vi "LOAD CELL READ.vi"(8 "error in (no error)":errorcluster, 11 "main ref":T1) -> (0 "error out":errorcluster)   [LabVIEW 2025]
uses:
  controls/LAB-IQ UI Data.ctl
  <vilib>/Analysis/baseanly.llb/Mean (DBL).vi
  <vilib>/Analysis/5stat.llb/RMS (DBL).vi
  <vilib>/Analysis/NI_AALBase.lvlib
  <vilib>/ptbypt/NI_PtbyPt.lvlib
  <vilib>/Analysis/NI_AALPro.lvlib
panel:
  out "Fload 3":dbl
  out "Fload 2":dbl
  out "Fload":dbl
  out "Friction":dbl
  out "Load Temp":dbl
  out "Zload":dbl
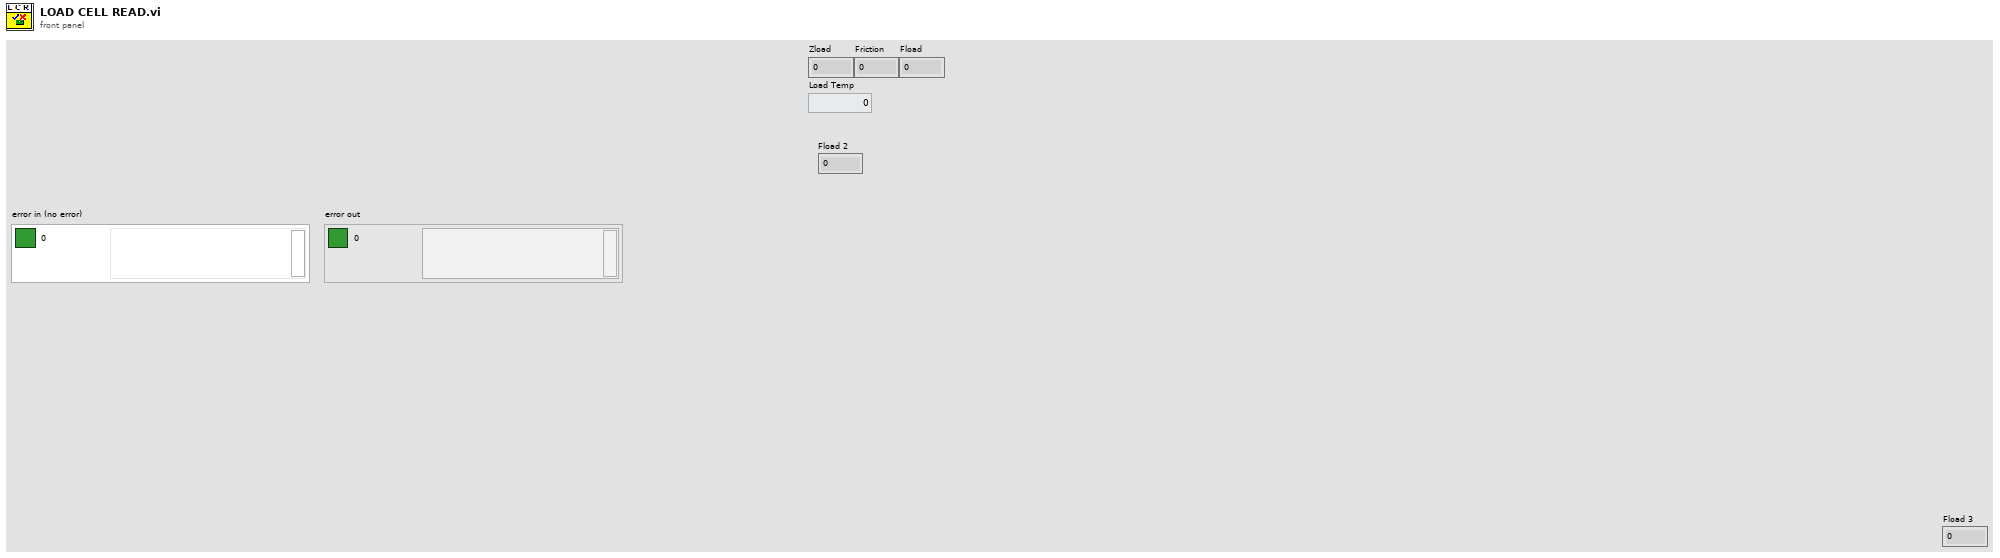
[diagram p1: front panel]
types:
  T1 = typedef "LAB-IQ UI Data.ctl" = cluster{"Main Home Screen":cluster{"GUI":refnum<vi>, "Platform Settings":refnum<vi>, "Configure":refnum<vi>, "Home":refnum<vi>, "EXIT":refnum<vi>, "service 2":refnum<vi>, "MainPage":refnum<vi>, "Analysis":refnum<vi>}, "Platform Settings":cluster{"mm/s  Surge":refnum<vi>, "Update Surge Speed":refnum<vi>, "Drive Error":refnum<vi>, "Disable Axis Jog Soft Limits":refnum<vi>, "mm/s  Sway":refnum<vi>, "Sway and Surge COM Status":refnum<vi>, "Heave COM Status":refnum<vi>, "Enable Platform":refnum<vi>, "Surge Forward Main":refnum<vi>, "Sway Right Main":refnum<vi>, "Sway Left Main":refnum<vi>, "Heave Down Main":refnum<vi>, "Heave Up main":refnum<vi>, "Update Sway Speed":refnum<vi>, "Update Heave Speed":refnum<vi>, "mm/s Heave":refnum<vi>, "mm/sec":refnum<vi>, "mm":refnum<vi>, "Surge Backward Main":refnum<vi>}, "Analysis Screen":cluster{"Analysis Home":refnum<vi>, "Surface Analysis":refnum<vi>, "Imaging":refnum<vi>, "Image Analysis":refnum<vi>, "Post Analysis":refnum<vi>}, "Config Screen":cluster{"Select Load Head":refnum<vi>, "Notes :":refnum<vi>, "FILE":refnum<vi>, "Sample ID :":refnum<vi>, "Operator ID :":refnum<vi>, "Operator Name :":refnum<vi>, "Auto":refnum<vi>}, "Motion Module":cluster{"zNL":refnum<vi>, "NL disp":refnum<vi>, "Rotary Tab":refnum<vi>, "Motion Direction:  3":refnum<vi>, "E.Velocity 2":refnum<vi>, "e.v/ssr 2":refnum<vi>, "Enter Fixed E.Velocity 2":refnum<vi>, "Enter Final SRR 2":refnum<vi>, "Enter initial SRR 2":refnum<vi>, "Enter Fixed SRR 2":refnum<vi>, "Enter the Final E.Velocity (m/s) 2":refnum<vi>, "Enter initial E.Velocity (m/s) 2":refnum<vi>, "Final Speed (RPM) 3":refnum<vi>, "Initial Speed (RPM) 2":refnum<vi>, "Enter the Final Velocity (m/s) 3":refnum<vi>, "Enter initial Velocity (m/s)  3":refnum<vi>, "Ramp Up 2":refnum<vi>, "TEST SELECTION":refnum<vi>, "SPEED SELECTION : ":refnum<vi>, "Angular Oscillation Set":refnum<vi>, "Traction":refnum<vi>, "Step Speed":refnum<vi>, "StepTable For Load-Speed":refnum<vi>, "StepTable For Speed":refnum<vi>, "Surge Forward MM":refnum<vi>, "Surge Backward MM":refnum<vi>, "M3 Image":refnum<vi>, "String 39":refnum<vi>, "Sway Left MM":refnum<vi>, "Sway Right MM":refnum<vi>, "Disable Axis Jog Soft Limits":refnum<vi>, "mm":refnum<vi>, "Heave Down MM":refnum<vi>, "Heave Up MM":refnum<vi>, "Wear Track Diameter (mm)":refnum<vi>, "Set WTD":refnum<vi>, "HomeScratch":refnum<vi>, "HomeRot":refnum<vi>, "PlaceModule":refnum<vi>, "Enter the Angle (Deg)":refnum<vi>, "Enter the Frequency (Hz)":refnum<vi>, "Motion Mode:":refnum<vi>, "LR Sway":refnum<vi>, "Rot Hor":refnum<vi>, "Scratch":refnum<vi>, "LR Cam":refnum<vi>, "MMBack":refnum<vi>, "MMNext":refnum<vi>, "Rot Ver":refnum<vi>, "Rotary Module Selection":refnum<vi>, "calculate rotary":refnum<vi>, "SPEED SELECTION : rotary":refnum<vi>, "Import 2":refnum<vi>, "Save 2":refnum<vi>, "File Path :  2":refnum<vi>, "String 45":refnum<vi>, "StepTable For Speed 3":refnum<vi>, "Enter the Speed(mm/sec)":refnum<vi>, "Enter the Speed(RPM)":refnum<vi>, "Enter Scratch Speed (mm/s):":refnum<vi>, "SwaySpeed Set":refnum<vi>, "Scartch Offset":refnum<vi>, "Motion type:":refnum<vi>, "HomeScratch 2":refnum<vi>, "Enter Scratch length (mm):":refnum<vi>, "Wear Track Diameter":refnum<vi>, "Rotary Speed Exced":refnum<vi>, "Scratch Mode":refnum<vi>, "No of Scratch":refnum<vi>}, "Environmental control":cluster{"Humidity  Status  3":refnum<vi>, "Low Temp  Status  2":refnum<vi>, "TK4 status 2":refnum<vi>, "Stage Temperature":refnum<vi>, "Sample Temperature":refnum<vi>, "Humidity (Amb)":refnum<vi>, "Clear List":refnum<vi>, "Add to list":refnum<vi>, "Wear":refnum<vi>, "Vibration":refnum<vi>, "Humidity (Chamber)":refnum<vi>, "Temperature (Chamber)":refnum<vi>, "ECR ":refnum<vi>, "Temperature (Amb)":refnum<vi>, "Microphone":refnum<vi>, "Acoustic Emission 3":refnum<vi>, "SNext":refnum<vi>, "APBack":refnum<vi>, "Enter the Temperature (°C):":refnum<vi>, "Enter the Stage \nTemperature (°C):":refnum<vi>, "Enter the Humidity (%Rh):":refnum<vi>, "Low Temp":refnum<vi>, "High Temp":refnum<vi>, "Humidity":refnum<vi>, "Sensors Picked":refnum<vi>}, "About Screen":cluster{"Password":refnum<vi>, "Home Service":refnum<vi>, "Advanced Setting":refnum<vi>, "About Tab":refnum<vi>, "ECR Port:":refnum<vi>, "Ramp Port:":refnum<vi>, "Installation/Replacement completed":refnum<vi>, "Loahead":refnum<vi>, "Heave and Surge COM Port:":refnum<vi>, "Sway COM Port:":refnum<vi>, "Temp Modbus:":refnum<vi>, "Humidity Port:":refnum<vi>, "Edit Gain Constants":refnum<vi>, "Save Gain Constants":refnum<vi>}, "Main Screen":cluster{"Main Screen Tab":refnum<vi>, "Angle and Frequency":refnum<vi>, "Stroke (mm)":refnum<vi>, "Angle (Deg)":refnum<vi>, "Main Speed Tab":refnum<vi>, "MTM MOTOR DISPLAY":refnum<vi>, "Disc Speed (m/sec)":refnum<vi>, "Ball Speed (m/sec)":refnum<vi>, "Disc Speed (RPM)":refnum<vi>, "Ball Speed (RPM)":refnum<vi>, "SPEED TAB":refnum<vi>, "Speed (m/sec)":refnum<vi>, "Set Speed (m/sec)":refnum<vi>, "Speed (RPM)":refnum<vi>, "Set Speed":refnum<vi>, "Time Tab":refnum<vi>, "Time ( HH:MM:SS ) 2":refnum<vi>, "Test Duration":refnum<vi>, "Test Duration 4":refnum<vi>, "TEST CYCLE":refnum<vi>, "TOTAL CYCLES":refnum<vi>, "Set Load (N)":refnum<vi>, "Temp Tabs":refnum<vi>, "Heater":refnum<vi>, "TK4 status":refnum<vi>, "ChamberTemp":refnum<vi>, "SetTmp":refnum<vi>, "Controller  Status":refnum<vi>, "ChamberTemp 2":refnum<vi>, "SetTmp 2":refnum<vi>, "Controller  Status 2":refnum<vi>, "ChamberTemp 3":refnum<vi>, "SetTmp 3":refnum<vi>, "Cooling":refnum<vi>, "Load Communication":refnum<vi>, "Ambient \nTemperature":refnum<vi>, "HumCOMStatus":refnum<vi>, "Ambient\n Humidity":refnum<vi>, "Freq (Hz)":refnum<vi>, "Load En":refnum<vi>, "NLt":refnum<vi>, "zNL 2":refnum<vi>, "Humidity On":refnum<vi>, "humidity disp":refnum<vi>, "Set Humidity":refnum<vi>, "NL disp 2":refnum<vi>, "Humidity On 2":refnum<vi>, "humidity disp 2":refnum<vi>, "Set Humidity 2":refnum<vi>, "NL disp 3":refnum<vi>, "AppLoadSeq scratch":refnum<vi>, "Stop Scratch":refnum<vi>, "ClrLog":refnum<vi>, "Trip Log":refnum<vi>, "STOP":refnum<vi>, "Start Test":refnum<vi>, "Test status":refnum<vi>, "AR Led":refnum<vi>, "Data":refnum<vi>, "Health":refnum<vi>, "Sway COM Status":refnum<vi>, "Heave COM Status":refnum<vi>, "Grp Tab":refnum<vi>, "Sub Graph":refnum<vi>, "SD (mm)":refnum<vi>, "Siliding distance Reset Graph":refnum<vi>, "SDGp":refnum<vi>, "Humidity Reset Graph":refnum<vi>, "HumrGp":refnum<vi>, "Acoustic Emission (mV)":refnum<vi>, "Aqucostic Reset Graph":refnum<vi>, "gACQUOS":refnum<vi>, "ECR RESET":refnum<vi>, "ECR":refnum<vi>, "Temperature Reset":refnum<vi>, "Acoustic Emission (mV) 2":refnum<vi>, "Aqucostic Reset Graph 2":refnum<vi>, "gACQUOS 2":refnum<vi>, "ECR RESET 2":refnum<vi>, "ECR 2":refnum<vi>, "Temperature Reset 2":refnum<vi>, "Temperature (deg c)":refnum<vi>, "Speed Reset Graph":refnum<vi>, "Speed Tab":refnum<vi>, "MTM DISC  SPEED":refnum<vi>, "MTM BALL SPEED":refnum<vi>, "speed mm/sec":refnum<vi>, "Hymidity":refnum<vi>, "Humidity Disable trip":refnum<vi>, "CoF Trip  2":refnum<vi>, "Depth Trip":refnum<vi>, "Weart Deapth":refnum<vi>, "Depth Reset Graph":refnum<vi>, "Weart":refnum<vi>, "Depthz":refnum<vi>, "Depth (µm)":refnum<vi>, "WearGp":refnum<vi>, "NL Trip 2":refnum<vi>, "Load pid":refnum<vi>, "Load Disable Trip":refnum<vi>, "Load Reset Graph":refnum<vi>, "NL Display 4":refnum<vi>, "Main Chart 3":refnum<vi>, "BACK":refnum<vi>, "Depth Trip 2":refnum<vi>, "COF TRIP ":refnum<vi>, "Friction Force (N)":refnum<vi>, "FF Reset Graph":refnum<vi>, "FF Disable Trip":refnum<vi>, "FF TRIP":refnum<vi>, "COF Disable Trip":refnum<vi>, "COF Reset Graph":refnum<vi>, "Start Test Temp":refnum<vi>, "zFF":refnum<vi>, "Friction Force (N) Graph":refnum<vi>, "Coefficient of Friction":refnum<vi>, "Scratch Start Test":refnum<vi>, "FF Tab":refnum<vi>, "Cyclic Friction Force (N)":refnum<vi>, "CZ FF":refnum<vi>, "Cyclic Friction Force (N) Graph":refnum<vi>, "Cyclic Coefficient of Friction":refnum<vi>, "Cyclic FF TRIP":refnum<vi>, "Cyclic FF Disable Trip":refnum<vi>, "cyclic COF Disable Trip":refnum<vi>, "cyclic COF TRIP":refnum<vi>, "cyclic COF Reset Graph":refnum<vi>, "Cyclic FF Reset Graph":refnum<vi>, "Test Trip":refnum<vi>, "Multi Scratch Pass":refnum<vi>, "Scratch Start Recording":refnum<vi>}, "Loading":cluster{"Indentation":refnum<vi>, "Reference Sample":refnum<vi>, "Load Cell Communication Slide":refnum<vi>, "com 3":refnum<vi>, "com":refnum<vi>, "DecaForce COM Status":refnum<vi>, "Update":refnum<vi>, "Clear 3":refnum<vi>, "seq":refnum<vi>, "Stribeck table":refnum<vi>, "Stribeck Table  For loading":refnum<vi>, "Loading Mode":refnum<vi>, "Enter the Final Load (N)":refnum<vi>, "Enter the CoF Trip":refnum<vi>, "Enter the Friction Force Trip":refnum<vi>, "Enter the Normal load Trip":refnum<vi>, "Enter the Load  (N)":refnum<vi>, "KiloForce":refnum<vi>, "DecaForce ":refnum<vi>, "MicroForce":refnum<vi>, "LHBack":refnum<vi>, "LHNext":refnum<vi>, "Enter the Loading Rate (N/min)":refnum<vi>, "Message":refnum<vi>, "Warning 2":refnum<vi>, "SSP 0.75":refnum<vi>, "SSP 0.5":refnum<vi>, "SSP 0.3":refnum<vi>, "Warning":refnum<vi>, "gui GIF":refnum<vi>, "Communication is established":refnum<vi>, "AppLoad 4":refnum<vi>, "Multipoint":refnum<vi>, "Load Selection":refnum<vi>}, "PID":cluster{"Ramp MulFac":refnum<vi>, "pulses LoadDiffRamp(2..10)":refnum<vi>, "PulseControlRamp(diff<=3N)":refnum<vi>, "SetLoadDeadband(%) Load(0-10N)":refnum<vi>, "PID gains out delay (microForce)":refnum<vi>, "Ramp":refnum<vi>, "Gain 2":refnum<vi>, "pulses LoadDiff(2..10)":refnum<vi>, "pulses LoadDiff(11..50)":refnum<vi>, "PulseControl(diff<=3N)":refnum<vi>, "SetLoadDeadband(%)  2":refnum<vi>, "Dummy Run":refnum<vi>, "Vertical load (N)":refnum<vi>, "AutoTune":refnum<vi>, "Offset 3 ":refnum<vi>, "apply load":refnum<vi>, "Offset  3":refnum<vi>, "apply load 2":refnum<vi>, "Enter ByPass Load":refnum<vi>, "reinit 3":refnum<vi>, "output range delay":refnum<vi>, "PID gains out delay":refnum<vi>, "Bypass Load":refnum<vi>, "pulsesSent":refnum<vi>, "pulses ":refnum<vi>, "actpid":refnum<vi>, "gFF Rot":refnum<vi>, "pulses LoadDiff(21..1000)":refnum<vi>, "Delay":refnum<vi>, "deadband":refnum<vi>}, "Config Parameters":cluster{"Tab Control 3":refnum<vi>, "Tab Control 19":refnum<vi>, "SAMPLES":refnum<vi>, "Re-initilaize":refnum<vi>, "Filter ON/OFF":refnum<vi>, "TracHomeSurgeOffsetCounts 10MM":refnum<vi>, "TracHomeSwayOffsetCounts 10MM":refnum<vi>, "Acoustic Emission:":refnum<vi>, "Apply Filter (FF)":refnum<vi>, "Filter% 2":refnum<vi>, "Apply Filter (Load)":refnum<vi>, "Filter% ":refnum<vi>, "Sway distance (mm)":refnum<vi>, "Surge distance (mm)":refnum<vi>, "DataSavingLoopDelay(ms)":refnum<vi>, "SAVE 2":refnum<vi>, "Enter Distance":refnum<vi>, "Sway Counts:":refnum<vi>, "Distance (mm): 3":refnum<vi>, "Surge Counts:":refnum<vi>, "Distance (mm): 2":refnum<vi>, "Distance (mm):":refnum<vi>, "Heave Counts:":refnum<vi>, "LRMHomeSurgeOffsetCounts":refnum<vi>, "LRMHomeSwayOffsetCounts":refnum<vi>, "TracHomeSurgeOffsetCounts 20MM":refnum<vi>, "TracHomeSwayOffsetCounts 20MM":refnum<vi>, "RotHomeSwayOffsetCounts":refnum<vi>, "RotHomeSurgeOffsetCounts":refnum<vi>, "Heave distance":refnum<vi>, "Zmm":refnum<vi>, "Heave Pulses/mm":refnum<vi>, "Surge Pulses/mm":refnum<vi>, "Sway Pulses/mm":refnum<vi>, "Heave Pitch":refnum<vi>, "Surge Pitch":refnum<vi>, "Sway Pitch":refnum<vi>, "Heave PPR":refnum<vi>, "Surge PPR":refnum<vi>, "Sway PPR":refnum<vi>, "Tab Control 5":refnum<vi>, "Tab Control 14":refnum<vi>, "Tab Control 26":refnum<vi>, "AE":refnum<vi>, "Heave Loop Delay":refnum<vi>, "Heave PID Speed":refnum<vi>, "Surge Jog Speed":refnum<vi>, "Heave Jog Speed":refnum<vi>, "Sway Loop Delay":refnum<vi>, "Sway PID Speed":refnum<vi>, "Sway Jog Speed":refnum<vi>, "DEPTH TRIP VALUE":refnum<vi>, "LOAD TRIP VALUE":refnum<vi>, "DEPTH TRIP   ENABLE":refnum<vi>, "LOAD TRIP  ENABLE":refnum<vi>, "CYCLIC FF TRIP VALUE":refnum<vi>, "FF TRIP VALUE":refnum<vi>, "CYCLIC CoF TRIP VALUE":refnum<vi>, "COF TRIP VALUE":refnum<vi>, "CYCLIC COF TRIP  ENABLE":refnum<vi>, "CYCLIC FF TRIP  ENABLE":refnum<vi>, "FF TRIP  ENABLE":refnum<vi>, "COF TRIP  ENABLE":refnum<vi>}, "Loading Com Port":cluster{"ClearAll":refnum<vi>, "Mz(Nm)":refnum<vi>, "My(Nm)":refnum<vi>, "Mx(Nm)":refnum<vi>, "Save Dwell":refnum<vi>, "Mx ":refnum<vi>, "My ":refnum<vi>, "Mz":refnum<vi>, "Fx(N)":refnum<vi>, "Fy(N)":refnum<vi>, "Fz(N)":refnum<vi>, "ZeroAll":refnum<vi>, "Acq Delay (ms)":refnum<vi>, "Burst Delay (ms)":refnum<vi>, "model":refnum<vi>, "SN":refnum<vi>, "FFx(N)":refnum<vi>, "Sensor IP":refnum<vi>, "Port":refnum<vi>, "FFy(N)":refnum<vi>, "Load(N)":refnum<vi>, "delete Handle":refnum<vi>, "Create Handle":refnum<vi>, "ft_data":refnum<vi>, "ft_range":refnum<vi>, "ft_data 2":refnum<vi>, "stop 6":refnum<vi>, "running_flag":refnum<vi>, "ft_udp_handle":refnum<vi>, "get-data-return":refnum<vi>, "get-range-return":refnum<vi>, "zero-return":refnum<vi>, "filter-return":refnum<vi>, "initial-return":refnum<vi>, "deleteHandle-result":refnum<vi>, "Load Cell Temp":refnum<vi>}, "Heave AND Surge":cluster{"SURGE POSE":refnum<vi>, "error out Read":refnum<vi>, "HEAVE POSE":refnum<vi>, "State":refnum<vi>, "Homed":refnum<vi>, "Sequence ID":refnum<vi>, "error out Write":refnum<vi>, "faultCode":refnum<vi>, "Ack ID":refnum<vi>, "SPEED":refnum<vi>, "Distance":refnum<vi>, "Mode Command":refnum<vi>, "Heave and Surge Read":refnum<vi>, "Read Heave Temp":refnum<vi>, "Spare 15":refnum<vi>, "Spare 14":refnum<vi>, "Spare 13":refnum<vi>, "Spare 12":refnum<vi>, "Spare 11":refnum<vi>, "Spare 10":refnum<vi>, "Spare 9":refnum<vi>, "Spare 8":refnum<vi>, "Spare 7":refnum<vi>, "Spare 6":refnum<vi>, "Spare 5":refnum<vi>, "Spare 4":refnum<vi>, "Spare 2":refnum<vi>, "Spare 1":refnum<vi>, "Node Id":refnum<vi>, "Spare 3":refnum<vi>, "SPARE 4":refnum<vi>, "SPARE 3":refnum<vi>, "SPARE 2":refnum<vi>, "SPARE 1":refnum<vi>, "fwMajor":refnum<vi>, "fwMinor":refnum<vi>, "Manual Write":refnum<vi>, "Heave and Surge Write":refnum<vi>}, "New PID LOGIC":cluster{"Fine Tune Zone":refnum<vi>, "PID SDelay":refnum<vi>, "Max_pos_limit":refnum<vi>, "Min_pos_limit":refnum<vi>, "i_limit":refnum<vi>, "pct_scale":refnum<vi>, "Deadband":refnum<vi>, "Kd":refnum<vi>, "Ki":refnum<vi>, "Kp":refnum<vi>, "Current Position":refnum<vi>, "Set Load":refnum<vi>, "Current Load":refnum<vi>, "Pulse delta":refnum<vi>, "Init Step":refnum<vi>, "Max Step Linit":refnum<vi>}, "SWAY ":cluster{"fwMajor":refnum<vi>, "Homed":refnum<vi>, "Rotary POSE":refnum<vi>, "State":refnum<vi>, "SWAY POSE":refnum<vi>, "Ack ID":refnum<vi>, "faultCode":refnum<vi>, "Node Id":refnum<vi>, "fwMinor":refnum<vi>, "Spare 6":refnum<vi>, "Spare 5":refnum<vi>, "Spare 4":refnum<vi>, "Spare 3":refnum<vi>, "Spare 2":refnum<vi>, "Spare 1":refnum<vi>, "Spare 7":refnum<vi>, "SPARE  5":refnum<vi>, "error out Write  SWAY ":refnum<vi>, "error out Read SWAY ":refnum<vi>, "Manual Write SWAY ":refnum<vi>, "SWAY WRITE":refnum<vi>, "SPARE  4":refnum<vi>, "SPARE  3":refnum<vi>, "SPARE 2":refnum<vi>, "SPARE 1":refnum<vi>, "Spare 15":refnum<vi>, "Spare 14":refnum<vi>, "Spare 13":refnum<vi>, "Spare 12":refnum<vi>, "Spare 11":refnum<vi>, "Spare 9":refnum<vi>, "Spare 8":refnum<vi>, "SPEED":refnum<vi>, "Distance":refnum<vi>, "Mode Command":refnum<vi>, "Sequence ID":refnum<vi>, "SWAY READ":refnum<vi>, "Spare 10":refnum<vi>, "Read SWAY Temp":refnum<vi>}, "Analysis Screen":cluster{"Analysis Home":refnum<vi>, "Refresh 2":refnum<vi>, "MEAN 4":refnum<vi>, "SD 4":refnum<vi>, "VARIANCE 4":refnum<vi>, "MEAN  3":refnum<vi>, "SD  3":refnum<vi>, "VARIANCE  3":refnum<vi>, "MEAN 2":refnum<vi>, "SD  2":refnum<vi>, "VARIANCE 2":refnum<vi>, "MEAN":refnum<vi>, "SD":refnum<vi>, "VARIANCE":refnum<vi>, "File 4 Discription":refnum<vi>, "OPEN 4":refnum<vi>, "File Name 4":refnum<vi>, "OPEN 3":refnum<vi>, "File 3 Discription":refnum<vi>, "File Name 3":refnum<vi>, "Y-AXIS":refnum<vi>, "X-AXIS":refnum<vi>, "XY Graph":refnum<vi>, "File Name 2":refnum<vi>, "File Name 1":refnum<vi>, "OPEN 2":refnum<vi>, "OPEN 1":refnum<vi>, "File 1 Discription ":refnum<vi>, "File 2 Discription":refnum<vi>, "Export":refnum<vi>, "File Format":refnum<vi>}}
  T2 = enum16{"INIT", "SETLOWPASSFILTER", "SETZERO", "GETSENSORINFO", "GETRANGE", "ZEROALL", "READDATA", "UNINITIAL", "DELETEHANDLE"}
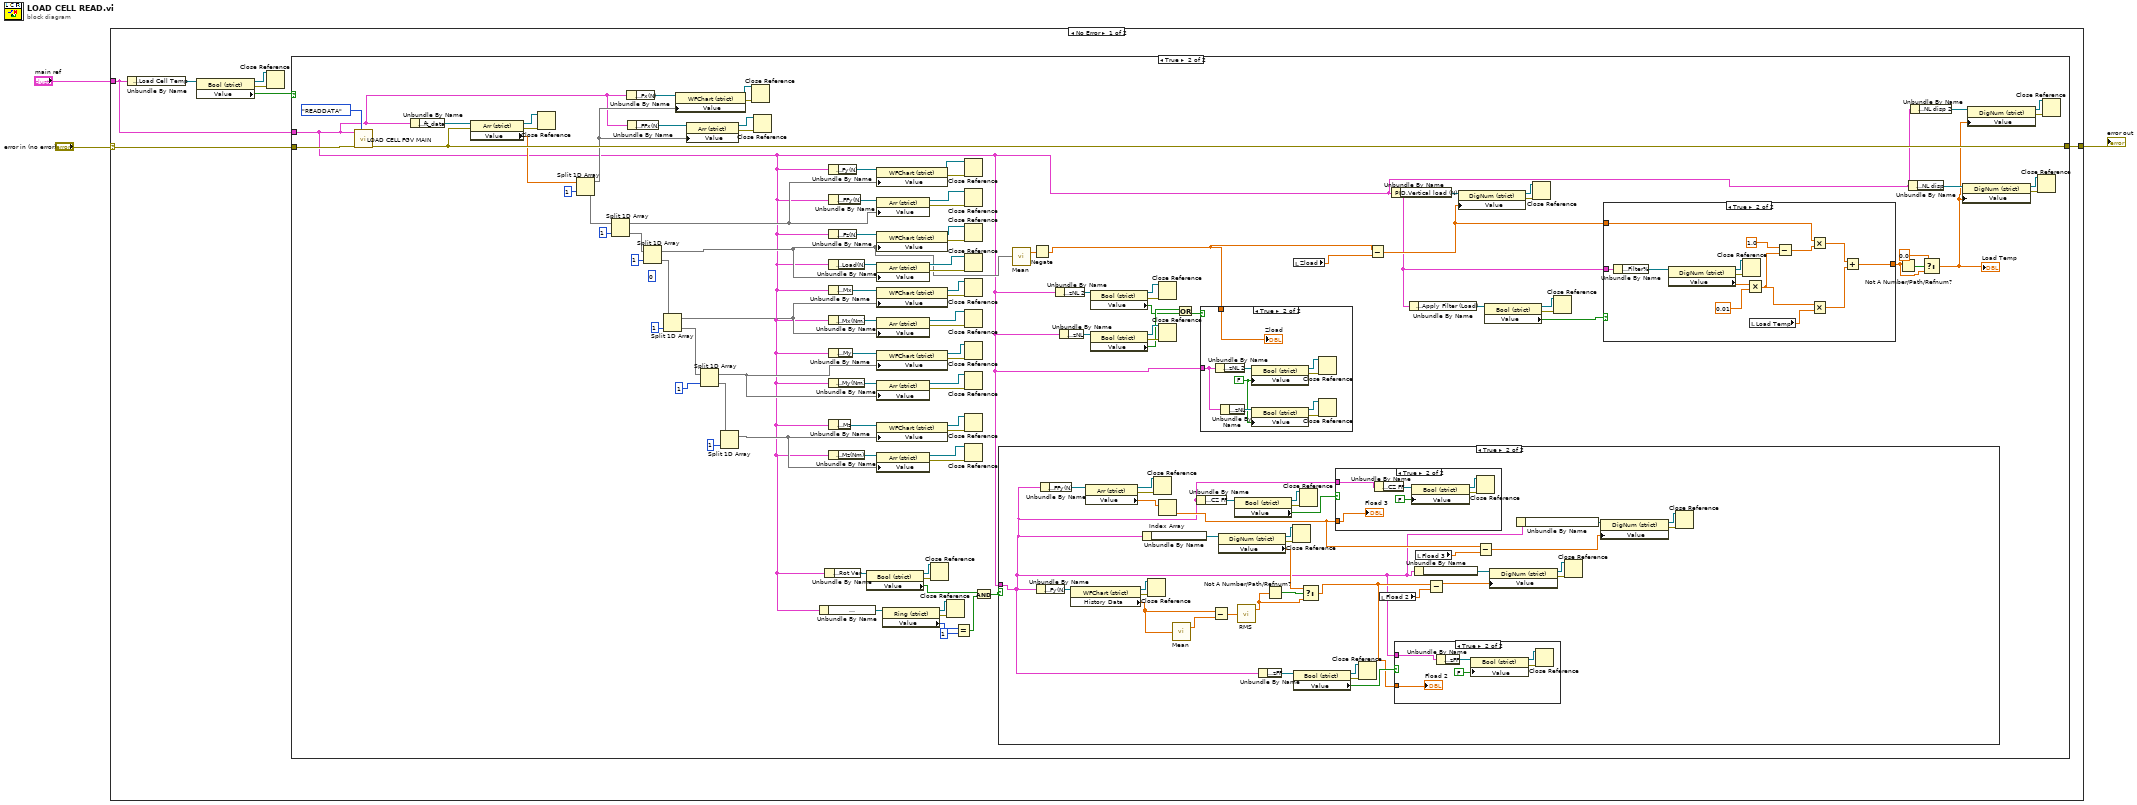
[diagram p0: block diagram]
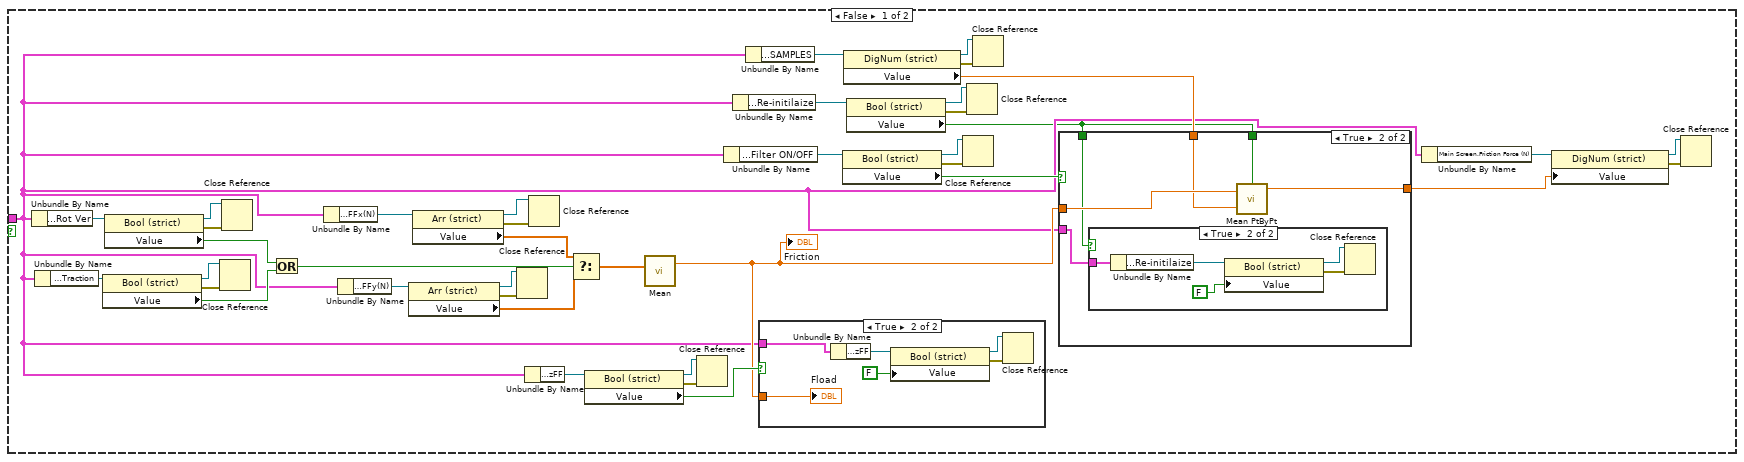
[diagram p3: hidden frame]
diagram:
  n1 = case shown="No Error" "error in (no error)" {
    selector: "error in (no error)" -> [w6 _]
    tunnel: "main ref" -> [w4 _]
    tunnel: [w5 _] -> w1
    frame No Error {
      n2 = Unbundle By Name(w4) -> ("Loading Com Port.Load Cell Temp"=w8:refnum<vi>)
      n3 = property class="Bool (strict)"(reference=w8) -> (reference out=w10:refnum<vi>, error out=w9:errorcluster, "Value"=w7:bool)  [unwired: 1 in]
      n4 = Close Reference(reference=w10, error in (no error)=w9) -> ()  [unwired: 1 out]
      n5 = case shown="True" w7 {
        tunnel: w6 -> [w11 w113]
        tunnel: [w11 w98] -> w5
        tunnel: w4 -> [_ w18]
        frame False {
        }
        frame True {
          (unwired) 0 ("index")
          n6 = call "LOAD CELL FGV MAIN.vi"("Enum"=T2."READDATA", "error in (no error)"=w113, "main ref"=w18) -> ("error IO"=w98:errorcluster)  [unwired: 8 in]
          n7 = Unbundle By Name(w18) -> ("Loading Com Port.ft_data"=w100:refnum<vi>)
          n8 = property class="Arr (strict)"(reference=w100, error in=w98) -> (reference out=w97:refnum<vi>, error out=w99:errorcluster, "Value"=w96:dbl[])
          n9 = Close Reference(reference=w97, error in (no error)=w99) -> ()  [unwired: 1 out]
          n10 = Split 1D Array(array=w96, index=1) -> (first subarray=w89:dbl[], second subarray=w111:dbl[])
          n11 = Split 1D Array(array=w111, index=1) -> (first subarray=w82:dbl[], second subarray=w107:dbl[])
          n12 = Unbundle By Name(w18) -> ("Loading Com Port.Fx(N)"=w95:refnum<vi>)
          n13 = Unbundle By Name(w18) -> ("Loading Com Port.FFx(N)"=w90:refnum<vi>)
          n14 = Split 1D Array(array=w107, index=1) -> (first subarray=w53:dbl[], second subarray=w103:dbl[])
          n15 = Split 1D Array(array=w103, index=1) -> (first subarray=w69:dbl[], second subarray=w102:dbl[])
          n16 = property class="WFChart (strict)"(reference=w95, "Value"=w89) -> (reference out=w93:refnum<vi>, error out=w94:errorcluster)  [unwired: 1 in]
          n17 = property class="Arr (strict)"(reference=w90, "Value"=w89) -> (reference out=w92:refnum<vi>, error out=w91:errorcluster)  [unwired: 1 in]
          n18 = Split 1D Array(array=w102, index=1) -> (first subarray=w62:dbl[], second subarray=w101:dbl[])
          n19 = Split 1D Array(array=w101, index=1) -> (first subarray=w55:dbl[])  [unwired: 1 out]
          n20 = Close Reference(reference=w93, error in (no error)=w94) -> ()  [unwired: 1 out]
          n21 = Close Reference(reference=w92, error in (no error)=w91) -> ()  [unwired: 1 out]
          n22 = Unbundle By Name(w18) -> ("Motion Module.Motion Mode:"=w17:refnum<vi>)
          n23 = Unbundle By Name(w18) -> ("Motion Module.Rot Ver"=w23:refnum<vi>)
          n24 = Unbundle By Name(w18) -> ("Loading Com Port.Fy(N)"=w88:refnum<vi>)
          n25 = Unbundle By Name(w18) -> ("Loading Com Port.FFy(N)"=w83:refnum<vi>)
          n26 = Unbundle By Name(w18) -> ("Loading Com Port.Fz(N)"=w76:refnum<vi>)
          n27 = Unbundle By Name(w18) -> ("Loading Com Port.Load(N)"=w81:refnum<vi>)
          n28 = Unbundle By Name(w18) -> ("Loading Com Port.Mx"=w75:refnum<vi>)
          n29 = Unbundle By Name(w18) -> ("Loading Com Port.Mx(Nm)"=w70:refnum<vi>)
          n30 = Unbundle By Name(w18) -> ("Loading Com Port.My"=w63:refnum<vi>)
          n31 = Unbundle By Name(w18) -> ("Loading Com Port.My(Nm)"=w68:refnum<vi>)
          n32 = Unbundle By Name(w18) -> ("Loading Com Port.Mz"=w61:refnum<vi>)
          n33 = Unbundle By Name(w18) -> ("Loading Com Port.Mz(Nm)"=w56:refnum<vi>)
          n34 = property class="Bool (strict)"(reference=w23) -> (reference out=w21:refnum<vi>, error out=w22:errorcluster, "Value"=w14:bool)  [unwired: 1 in]
          n35 = property class="WFChart (strict)"(reference=w88, "Value"=w82) -> (reference out=w86:refnum<vi>, error out=w87:errorcluster)  [unwired: 1 in]
          n36 = property class="Arr (strict)"(reference=w83, "Value"=w82) -> (reference out=w85:refnum<vi>, error out=w84:errorcluster)  [unwired: 1 in]
          n37 = property class="WFChart (strict)"(reference=w76, "Value"=w53) -> (reference out=w78:refnum<vi>, error out=w77:errorcluster)  [unwired: 1 in]
          n38 = property class="Arr (strict)"(reference=w81, "Value"=w53) -> (reference out=w79:refnum<vi>, error out=w80:errorcluster)  [unwired: 1 in]
          n39 = property class="WFChart (strict)"(reference=w75, "Value"=w69) -> (reference out=w73:refnum<vi>, error out=w74:errorcluster)  [unwired: 1 in]
          n40 = property class="Arr (strict)"(reference=w70, "Value"=w69) -> (reference out=w72:refnum<vi>, error out=w71:errorcluster)  [unwired: 1 in]
          n41 = property class="WFChart (strict)"(reference=w63, "Value"=w62) -> (reference out=w65:refnum<vi>, error out=w64:errorcluster)  [unwired: 1 in]
          n42 = property class="Arr (strict)"(reference=w68, "Value"=w62) -> (reference out=w66:refnum<vi>, error out=w67:errorcluster)  [unwired: 1 in]
          n43 = property class="WFChart (strict)"(reference=w61, "Value"=w55) -> (reference out=w59:refnum<vi>, error out=w60:errorcluster)  [unwired: 1 in]
          n44 = property class="Arr (strict)"(reference=w56, "Value"=w55) -> (reference out=w58:refnum<vi>, error out=w57:errorcluster)  [unwired: 1 in]
          n45 = property class="Ring (strict)"(reference=w17) -> (reference out=w20:refnum<vi>, error out=w19:errorcluster, "Value"=w16:u16)  [unwired: 1 in]
          n46 = Close Reference(reference=w21, error in (no error)=w22) -> ()  [unwired: 1 out]
          n47 = Close Reference(reference=w20, error in (no error)=w19) -> ()  [unwired: 1 out]
          n48 = Equal?(x=w16, y=u16 1) -> (x = y?=w13:bool)
          n49 = Close Reference(reference=w86, error in (no error)=w87) -> ()  [unwired: 1 out]
          n50 = Close Reference(reference=w85, error in (no error)=w84) -> ()  [unwired: 1 out]
          n51 = Close Reference(reference=w78, error in (no error)=w77) -> ()  [unwired: 1 out]
          n52 = Close Reference(reference=w79, error in (no error)=w80) -> ()  [unwired: 1 out]
          n53 = Close Reference(reference=w73, error in (no error)=w74) -> ()  [unwired: 1 out]
          n54 = Close Reference(reference=w72, error in (no error)=w71) -> ()  [unwired: 1 out]
          n55 = Close Reference(reference=w65, error in (no error)=w64) -> ()  [unwired: 1 out]
          n56 = Close Reference(reference=w66, error in (no error)=w67) -> ()  [unwired: 1 out]
          n57 = Close Reference(reference=w59, error in (no error)=w60) -> ()  [unwired: 1 out]
          n58 = Close Reference(reference=w58, error in (no error)=w57) -> ()  [unwired: 1 out]
          n59 = And(x=w14, y=w13) -> (x .and. y?=w12:bool)
          n60 = case shown="True" w12 {
            tunnel: w18 -> [w116 w174]
            frame False {
              n61 = Unbundle By Name(w116) -> ("Motion Module.Rot Ver"=w146:refnum<vi>)
              n62 = Unbundle By Name(w116) -> ("Motion Module.Traction"=w151:refnum<vi>)
              n63 = property class="Bool (strict)"(reference=w151) -> (reference out=w149:refnum<vi>, error out=w150:errorcluster, "Value"=w153:bool)  [unwired: 1 in]
              n64 = property class="Bool (strict)"(reference=w146) -> (reference out=w148:refnum<vi>, error out=w147:errorcluster, "Value"=w152:bool)  [unwired: 1 in]
              n65 = Close Reference(reference=w149, error in (no error)=w150) -> ()  [unwired: 1 out]
              n66 = Close Reference(reference=w148, error in (no error)=w147) -> ()  [unwired: 1 out]
              n67 = Or(x=w152, y=w153) -> (x .or. y?=w137:bool)
              n68 = Unbundle By Name(w116) -> ("Loading Com Port.FFx(N)"=w143:refnum<vi>)
              n69 = Unbundle By Name(w116) -> ("Loading Com Port.FFy(N)"=w140:refnum<vi>)
              n70 = property class="Arr (strict)"(reference=w140) -> (reference out=w142:refnum<vi>, error out=w141:errorcluster, "Value"=w138:dbl[])  [unwired: 1 in]
              n71 = property class="Arr (strict)"(reference=w143) -> (reference out=w145:refnum<vi>, error out=w144:errorcluster, "Value"=w139:dbl[])  [unwired: 1 in]
              n72 = Close Reference(reference=w142, error in (no error)=w141) -> ()  [unwired: 1 out]
              n73 = Unbundle By Name(w116) -> ("Main Screen.zFF"=w135:refnum<vi>)
              n74 = Close Reference(reference=w145, error in (no error)=w144) -> ()  [unwired: 1 out]
              n75 = Select(t=w139, s=w137, f=w138) -> (s? t:f=w136:dbl[])
              n76 = property class="Bool (strict)"(reference=w135) -> (reference out=w133:refnum<vi>, error out=w134:errorcluster, "Value"=w132:bool)  [unwired: 1 in]
              n77 = call-poly <vilib>:"Mean.vi"("X"=w136) -> ("mean"=w124:dbl)  [unwired: 1 out]
              "Friction" <- w124
              n78 = Close Reference(reference=w133, error in (no error)=w134) -> ()  [unwired: 1 out]
              n79 = Unbundle By Name(w116) -> ("Config Parameters.Filter ON/OFF"=w131:refnum<vi>)
              n80 = Unbundle By Name(w116) -> ("Config Parameters.Re-initilaize"=w125:refnum<vi>)
              n81 = Unbundle By Name(w116) -> ("Config Parameters.SAMPLES"=w123:refnum<vi>)
              n82 = case shown="True" w132 {
                tunnel: w116 -> [_ w168]
                tunnel: w124 -> [_ w166]
                frame False {
                }
                frame True {
                  n83 = Unbundle By Name(w168) -> ("Main Screen.zFF"=w169:refnum<vi>)
                  n84 = property class="Bool (strict)"(reference=w169, "Value"=FALSE) -> (reference out=w171:refnum<vi>, error out=w170:errorcluster)  [unwired: 1 in]
                  n85 = Close Reference(reference=w171, error in (no error)=w170) -> ()  [unwired: 1 out]
                  "Fload" <- w166
                }
              }
              n86 = property class="Bool (strict)"(reference=w131) -> (reference out=w129:refnum<vi>, error out=w130:errorcluster, "Value"=w128:bool)  [unwired: 1 in]
              n87 = property class="DigNum (strict)"(reference=w123) -> (reference out=w121:refnum<vi>, error out=w122:errorcluster, "Value"=w120:dbl)  [unwired: 1 in]
              n88 = property class="Bool (strict)"(reference=w125) -> (reference out=w127:refnum<vi>, error out=w126:errorcluster, "Value"=w114:bool)  [unwired: 1 in]
              n89 = Close Reference(reference=w129, error in (no error)=w130) -> ()  [unwired: 1 out]
              n90 = Close Reference(reference=w127, error in (no error)=w126) -> ()  [unwired: 1 out]
              n91 = Close Reference(reference=w121, error in (no error)=w122) -> ()  [unwired: 1 out]
              n92 = case shown="True" w128 {
                tunnel: w114 -> [_ w160]
                tunnel: w116 -> [_ w159]
                tunnel: w124 -> [w154 w158]
                tunnel: w120 -> [_ w157]
                tunnel: [w154 w156] -> w115
                tunnel: w114 -> [_ w155]
                frame False {
                }
                frame True {
                  n93 = case shown="True" w155 {
                    tunnel: w159 -> [_ w162]
                    frame False {
                    }
                    frame True {
                      n94 = Unbundle By Name(w162) -> ("Config Parameters.Re-initilaize"=w165:refnum<vi>)
                      n95 = property class="Bool (strict)"(reference=w165, "Value"=FALSE) -> (reference out=w163:refnum<vi>, error out=w164:errorcluster)  [unwired: 1 in]
                      n96 = Close Reference(reference=w163, error in (no error)=w164) -> ()  [unwired: 1 out]
                    }
                  }
                  n97 = call <vilib>:"Mean PtByPt.vi"("x"=w158, "sample length"=w157, "initialize"=w160) -> ("mean"=w156:dbl)  [unwired: 1 in, 1 out]
                }
              }
              n98 = Unbundle By Name(w116) -> ("Main Screen.Friction Force (N)"=w117:refnum<vi>)
              n99 = property class="DigNum (strict)"(reference=w117, "Value"=w115) -> (reference out=w119:refnum<vi>, error out=w118:errorcluster)  [unwired: 1 in]
              n100 = Close Reference(reference=w119, error in (no error)=w118) -> ()  [unwired: 1 out]
            }
            frame True {
              n101 = Unbundle By Name(w174) -> ("Loading Com Port.Fy(N)"=w208:refnum<vi>)
              n102 = Unbundle By Name(w174) -> ("Loading Com Port.FFy(N)"=w186:refnum<vi>)
              n103 = property class="WFChart (strict)"(reference=w208) -> (reference out=w206:refnum<vi>, error out=w207:errorcluster, "History Data"=w204:dbl[])  [unwired: 1 in]
              n104 = property class="Arr (strict)"(reference=w186) -> (reference out=w184:refnum<vi>, error out=w185:errorcluster, "Value"=w183:dbl[])  [unwired: 1 in]
              n105 = Unbundle By Name(w174) -> ("Main Screen.Friction Force (N)"=w195:refnum<vi>)
              n106 = Close Reference(reference=w206, error in (no error)=w207) -> ()  [unwired: 1 out]
              n107 = Close Reference(reference=w184, error in (no error)=w185) -> ()  [unwired: 1 out]
              n108 = Index Array(array=w183) -> (element=w177:dbl)  [unwired: 1 in]
              n109 = call-poly <vilib>:"Mean.vi"("X"=w204) -> ("mean"=w205:dbl)  [unwired: 1 out]
              n110 = Unbundle By Name(w174) -> ("Main Screen.CZ FF"=w182:refnum<vi>)
              n111 = Subtract(x=w204, y=w205) -> (x-y=w203:dbl[])
              n112 = property class="DigNum (strict)"(reference=w195) -> (reference out=w197:refnum<vi>, error out=w196:errorcluster, "Value"=w194:dbl)  [unwired: 1 in]
              n113 = property class="Bool (strict)"(reference=w182) -> (reference out=w180:refnum<vi>, error out=w181:errorcluster, "Value"=w179:bool)  [unwired: 1 in]
              n114 = call-poly <vilib>:"RMS.vi"("X"=w203) -> ("rms value"=w201:dbl)  [unwired: 1 out]
              n115 = Unbundle By Name(w174) -> ("Main Screen.zFF"=w193:refnum<vi>)
              n116 = Not A Number/Path/Refnum?(number/path/refnum=w201) -> (NaN/Path/Refnum?=w202:bool)
              n117 = Close Reference(reference=w197, error in (no error)=w196) -> ()  [unwired: 1 out]
              n118 = property class="Bool (strict)"(reference=w193) -> (reference out=w191:refnum<vi>, error out=w192:errorcluster, "Value"=w190:bool)  [unwired: 1 in]
              n119 = Close Reference(reference=w180, error in (no error)=w181) -> ()  [unwired: 1 out]
              n120 = Select(t=w194, s=w202, f=w201) -> (s? t:f=w189:dbl)
              n121 = case shown="True" w179 {
                tunnel: w174 -> [_ w211]
                tunnel: w177 -> [_ w209]
                frame False {
                }
                frame True {
                  n122 = Unbundle By Name(w211) -> ("Main Screen.CZ FF"=w212:refnum<vi>)
                  n123 = property class="Bool (strict)"(reference=w212, "Value"=FALSE) -> (reference out=w214:refnum<vi>, error out=w213:errorcluster)  [unwired: 1 in]
                  n124 = Close Reference(reference=w214, error in (no error)=w213) -> ()  [unwired: 1 out]
                  "Fload 3" <- w209
                }
              }
              n125 = Close Reference(reference=w191, error in (no error)=w192) -> ()  [unwired: 1 out]
              n126 = local read "Fload 2"() -> (w187:dbl)
              n127 = case shown="True" w190 {
                tunnel: w174 -> [_ w217]
                tunnel: w189 -> [_ w215]
                frame False {
                }
                frame True {
                  n128 = Unbundle By Name(w217) -> ("Main Screen.zFF"=w218:refnum<vi>)
                  n129 = property class="Bool (strict)"(reference=w218, "Value"=FALSE) -> (reference out=w220:refnum<vi>, error out=w219:errorcluster)  [unwired: 1 in]
                  n130 = Close Reference(reference=w220, error in (no error)=w219) -> ()  [unwired: 1 out]
                  "Fload 2" <- w215
                }
              }
              n131 = Unbundle By Name(w174) -> ("Main Screen.Friction Force (N)"=w198:refnum<vi>)
              n132 = local read "Fload 3"() -> (w178:dbl)
              n133 = Subtract(x=w189, y=w187) -> (x-y=w188:dbl)
              n134 = Subtract(x=w177, y=w178) -> (x-y=w172:dbl)
              n135 = property class="DigNum (strict)"(reference=w198, "Value"=w188) -> (reference out=w200:refnum<vi>, error out=w199:errorcluster)  [unwired: 1 in]
              n136 = Unbundle By Name(w174) -> ("Main Screen.Cyclic Friction Force (N)"=w175:refnum<vi>)
              n137 = Close Reference(reference=w200, error in (no error)=w199) -> ()  [unwired: 1 out]
              n138 = property class="DigNum (strict)"(reference=w175, "Value"=w172) -> (reference out=w173:refnum<vi>, error out=w176:errorcluster)  [unwired: 1 in]
              n139 = Close Reference(reference=w173, error in (no error)=w176) -> ()  [unwired: 1 out]
            }
          }
          n140 = call-poly <vilib>:"Mean.vi"("X"=w53) -> ("mean"=w54:dbl)  [unwired: 1 out]
          n141 = Negate(x=w54) -> (-x=w40:dbl)
          n142 = Unbundle By Name(w18) -> ("Main Screen.zNL 2"=w44:refnum<vi>)
          n143 = Unbundle By Name(w18) -> ("Motion Module.zNL"=w49:refnum<vi>)
          n144 = property class="Bool (strict)"(reference=w44) -> (reference out=w46:refnum<vi>, error out=w45:errorcluster, "Value"=w42:bool)  [unwired: 1 in]
          n145 = property class="Bool (strict)"(reference=w49) -> (reference out=w47:refnum<vi>, error out=w48:errorcluster, "Value"=w43:bool)  [unwired: 1 in]
          n146 = Close Reference(reference=w46, error in (no error)=w45) -> ()  [unwired: 1 out]
          n147 = Close Reference(reference=w47, error in (no error)=w48) -> ()  [unwired: 1 out]
          n148 = Or(x=w43, y=w42) -> (x .or. y?=w41:bool)
          n149 = case shown="True" w41 {
            tunnel: w40 -> [_ w244]
            tunnel: w18 -> [_ w237]
            frame False {
            }
            frame True {
              w236 = FALSE ("Value")
              n150 = Unbundle By Name(w237) -> ("Main Screen.zNL 2"=w238:refnum<vi>)
              n151 = Unbundle By Name(w237) -> ("Motion Module.zNL"=w243:refnum<vi>)
              n152 = property class="Bool (strict)"(reference=w238, "Value"=w236) -> (reference out=w240:refnum<vi>, error out=w239:errorcluster)  [unwired: 1 in]
              n153 = property class="Bool (strict)"(reference=w243, "Value"=w236) -> (reference out=w241:refnum<vi>, error out=w242:errorcluster)  [unwired: 1 in]
              n154 = Close Reference(reference=w240, error in (no error)=w239) -> ()  [unwired: 1 out]
              n155 = Close Reference(reference=w241, error in (no error)=w242) -> ()  [unwired: 1 out]
              "Zload" <- w244
            }
          }
          n156 = local read "Zload"() -> (w39:dbl)
          n157 = Subtract(x=w40, y=w39) -> (x-y=w34:dbl)
          n158 = Unbundle By Name(w18) -> ("PID.Vertical load (N)"=w52:refnum<vi>)
          n159 = Unbundle By Name(w18) -> ("Config Parameters.Apply Filter (Load)"=w36:refnum<vi>)
          n160 = property class="DigNum (strict)"(reference=w52, "Value"=w34) -> (reference out=w50:refnum<vi>, error out=w51:errorcluster)  [unwired: 1 in]
          n161 = property class="Bool (strict)"(reference=w36) -> (reference out=w38:refnum<vi>, error out=w37:errorcluster, "Value"=w35:bool)  [unwired: 1 in]
          n162 = Close Reference(reference=w50, error in (no error)=w51) -> ()  [unwired: 1 out]
          n163 = Close Reference(reference=w38, error in (no error)=w37) -> ()  [unwired: 1 out]
          n164 = case shown="True" w35 {
            tunnel: w18 -> [_ w232]
            tunnel: w34 -> [w221 w226]
            tunnel: [w221 w223] -> w31
            frame False {
            }
            frame True {
              n165 = Unbundle By Name(w232) -> ("Config Parameters.Filter%"=w235:refnum<vi>)
              n166 = property class="DigNum (strict)"(reference=w235) -> (reference out=w233:refnum<vi>, error out=w234:errorcluster, "Value"=w231:dbl)  [unwired: 1 in]
              n167 = Close Reference(reference=w233, error in (no error)=w234) -> ()  [unwired: 1 out]
              n168 = Multiply(x=w231, y=0.01) -> (x*y=w228:dbl)
              n169 = local read "Load Temp"() -> (w222:dbl)
              n170 = Subtract(x=1.0, y=w228) -> (x-y=w227:dbl)
              n171 = Multiply(x=w226, y=w227) -> (x*y=w225:dbl)
              n172 = Multiply(x=w228, y=w222) -> (x*y=w224:dbl)
              n173 = Add(x=w225, y=w224) -> (x+y=w223:dbl)
            }
          }
          n174 = Not A Number/Path/Refnum?(number/path/refnum=w31) -> (NaN/Path/Refnum?=w33:bool)
          n175 = Unbundle By Name(w18) -> ("Motion Module.NL disp"=w28:refnum<vi>)
          n176 = Unbundle By Name(w18) -> ("Main Screen.NL disp 2"=w27:refnum<vi>)
          n177 = Select(t=0.0, s=w33, f=w31) -> (s? t:f=w24:dbl)
          "Load Temp" <- w24
          n178 = property class="DigNum (strict)"(reference=w28, "Value"=w24) -> (reference out=w30:refnum<vi>, error out=w29:errorcluster)  [unwired: 1 in]
          n179 = property class="DigNum (strict)"(reference=w27, "Value"=w24) -> (reference out=w25:refnum<vi>, error out=w26:errorcluster)  [unwired: 1 in]
          n180 = Close Reference(reference=w30, error in (no error)=w29) -> ()  [unwired: 1 out]
          n181 = Close Reference(reference=w25, error in (no error)=w26) -> ()  [unwired: 1 out]
        }
      }
    }
    frame Error {
    }
  }
  "error out" <- w1
